vi "实验 1 子程序.vi"(1 "数值 3":dbl, 2 "数值 2":dbl, 3 "数值1":dbl) -> (0 "结果":dbl)   [LabVIEW 2017]
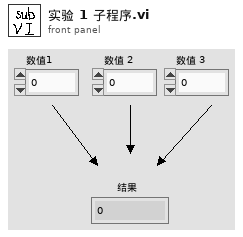
[diagram p1: front panel]
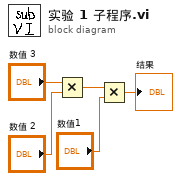
[diagram p0: block diagram]
diagram:
  n1 = Multiply(x="数值 3", y="数值 2") -> (x*y=w3:dbl)
  n2 = Multiply(x=w3, y="数值1") -> (x*y=→"结果":dbl)
